vi "XNET Read (State FlexRay Cycle Macrotick).vi"(0 "session in":refnum<k21>, 11 "error in (no error)":errorcluster) -> (4 "session out":refnum<k21>, 6 "cycle":u8, 8 "macrotick":u16, 15 "error out":errorcluster)   [LabVIEW 2018]
doc: "Reads the current FlexRay global time using an XNET session."
uses:
  nixlvapi.dll
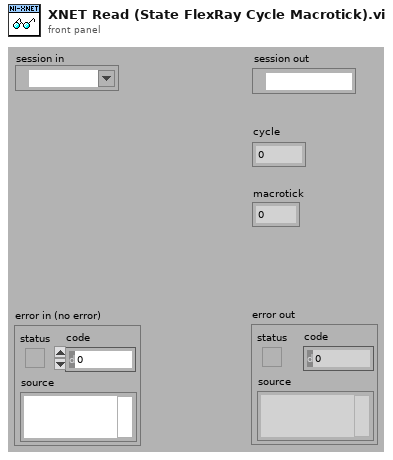
[diagram p1: front panel]
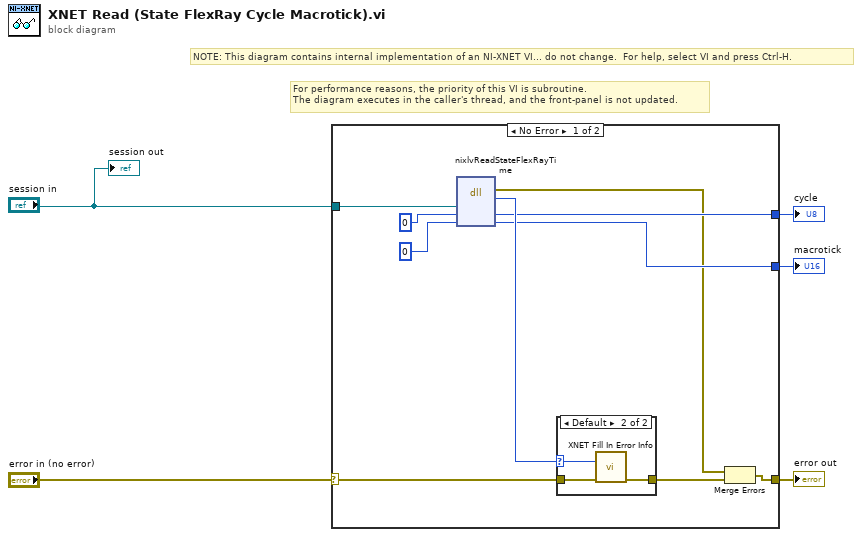
[diagram p0: block diagram]
diagram:
  # "For performance reasons, the priority of this VI is subroutine.\nThe diagram executes in the caller's thread, and the front-panel is not updated."
  # "NOTE: This diagram contains internal implementation of an NI-XNET VI... do not change.  For help, select VI and press Ctrl-H."
  n1 = case shown="No Error" "error in (no error)" {
    selector: "error in (no error)" -> [w14 w20]
    tunnel: "session in" -> [w15 _]
    tunnel: [w7 w20] -> w5
    tunnel: [w9 _] -> w2
    tunnel: [w8 _] -> w1
    frame No Error {
      n2 = dll-call lib="nixlvapi.*" fn="nixlvReadStateFlexRayTime"("sessionRef"=w15, "cycle"=u8 0 ("Cycle"), "macrotick"=u16 0 ("Macrotick")) -> (error out=w6:errorcluster, "return type"=w12:i32, "cycle"=w9:u8, "macrotick"=w8:u16)  [unwired: 3 in, 2 out]
      n3 = case shown="Default" w12 {
        selector: w12 -> [_ w17]
        tunnel: w14 -> [w16 w18]
        tunnel: [w16 w19] -> w13
        frame 0 {
        }
        frame Default {
          n4 = call "XNET Fill In Error Info.vi"("status code"=w17, "error in"=w18) -> ("error out"=w19:errorcluster)  [unwired: 13 out]
        }
      }
      n5 = Merge Errors(w6, w13) -> (w7:errorcluster)
    }
    frame Error {
    }
  }
  "error out" <- w5
  "macrotick" <- w1
  "cycle" <- w2
  "session out" <- "session in"
